vi "Y Axis Output WFM Graph.vi"(8 "error in (no error)":errorcluster, 10 "Y Axis Out":T1 caption="Enum", 11 "WaveformGraph in":refnum<vi>) -> (0 "error out":errorcluster)   [LabVIEW 2020, in "Instrument.Lockin.UI.lvclass"]
uses:
  Instrument.Lockin.UI.lvclass
  Typedefs/Y Axis Output-Enum.ctl
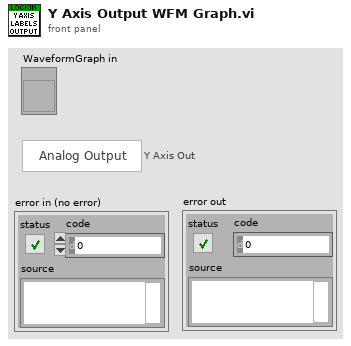
[diagram p1: front panel]
types:
  T1 = typedef "Instrument.Lockin.UI.lvclass/Y Axis Output-Enum.ctl" = enum16{"Analog Output", "Reference"}
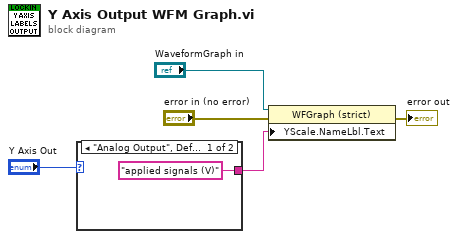
[diagram p0: block diagram]
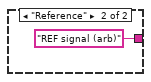
[diagram p2: hidden frame]
diagram:
  n1 = case shown="\"Analog Output\", Default" "Y Axis Out" {
    tunnel: ["applied signals (V)" ("Y Scale.Name Label.Text") "REF signal (arb)" ("Y Scale.Name Label.Text")] -> w1
    frame "Analog Output", Default {
    }
    frame "Reference" {
    }
  }
  n2 = property on="Property Node" class="WFGraph (strict)"(reference="WaveformGraph in", error in="error in (no error)", "YScale.NameLbl.Text"=w1) -> (error out=→"error out":errorcluster)  [unwired: 1 out]
